vi "micro2.vi"(8 "errin":errorcluster caption="constante d'erreur", 11 "offset%":dbl) -> (0 "errout":errorcluster caption="constante d'erreur")   [LabVIEW 2020]
uses:
  ctrl glo/VG_progressBar.vi
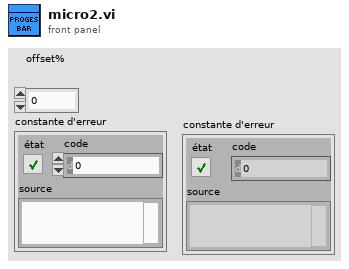
[diagram p1: front panel]
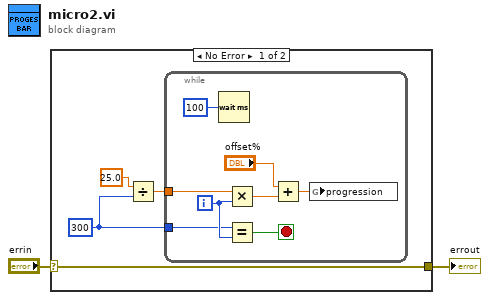
[diagram p0: block diagram]
diagram:
  n1 = case shown="No Error" "errin" {
    selector: "errin" -> [w3 w15]
    tunnel: [w3 w15] -> w1
    frame No Error {
      w4 = 300 ("x")
      n2 = Divide(x=25.0, y=w4) -> (x/y=w5:dbl)
      n3 = while {
        tunnel: w5 -> [w8]
        tunnel: w4 -> [w7]
        i -> [w9]
        stop <- w13 stop-if-true
        n4 = Wait (ms)(milliseconds to wait=u32 100 ("attente (ms)")) -> ()  [unwired: 1 out]
        n5 = Multiply(x=w8, y=w9) -> (x*y=w10:dbl)
        n6 = Equal?(x=w7, y=w9) -> (x = y?=w13:bool)
        n7 = Add(x="offset%", y=w10) -> (x+y=w12:dbl)
        n8 = global write "VG_progressBar.vi" "progression"(w12) -> ()
      }
    }
    frame Error {
    }
  }
  "errout" <- w1
